vi "AnyThingToDoubleArray.vi"(0 "Claster":variant, 5 "Prefix":string, 11 "error in (no error)":errorcluster) -> (4 "NAME_ARR":string[](array[string]), 6 "DBL_ARR":dbl[](array[numeric]), 15 "error out":errorcluster)   [LabVIEW 2019]
uses:
  <vilib>/Utility/error.llb/Error Cluster From Error Code.vi
  <vilib>/ErrorRing/Error Ring.xnode
  <vilib>/Utility/Data Type/Type Definitions/Data Type.ctl
  <vilib>/Utility/Data Type/NI_Data Type.lvlib
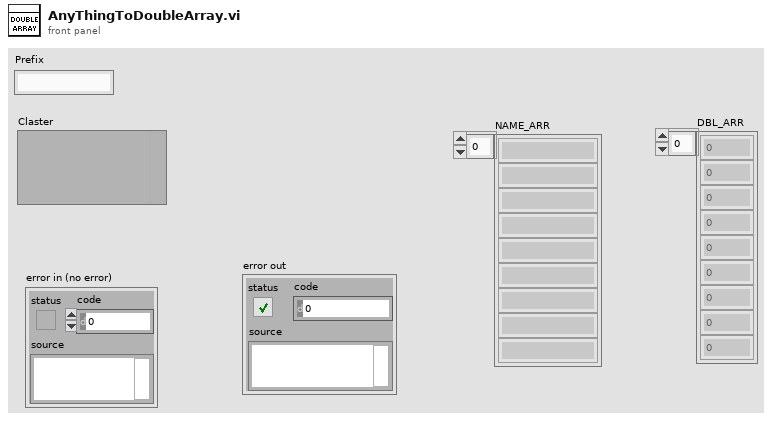
[diagram p1: front panel]
types:
  T1 = typedef "NI_Data Type.lvlib/Data Type.ctl" = enum8{"Invalid Type", "Void", "I8", "I16", "I32", "I64", "U8", "U16", "U32", "U64", "Single Float", "Double Float", "Extended Float", "Single Complex", "Double Complex", "Extended Complex", "Enum U8", "Enum U16", "Enum U32", "Enum U64", "Single Float With Unit", "Double Float With Unit", "Extended Float With Unit", "Single Complex with Unit", "Double Complex with Unit", "Extended Complex with Unit", "Boolean", "String", "Path", "Picture", "Tag", "Array", "Cluster", "Variant", "LV Variant", "Waveform", "Timestamp", "Digital Waveform", "Digital Data", "ExpressData", "Refnum", "External Data", "VI", "Poly VI", "LabVIEW Class Instance", "Fixed Point", "Set Collection", "Map Collection"}
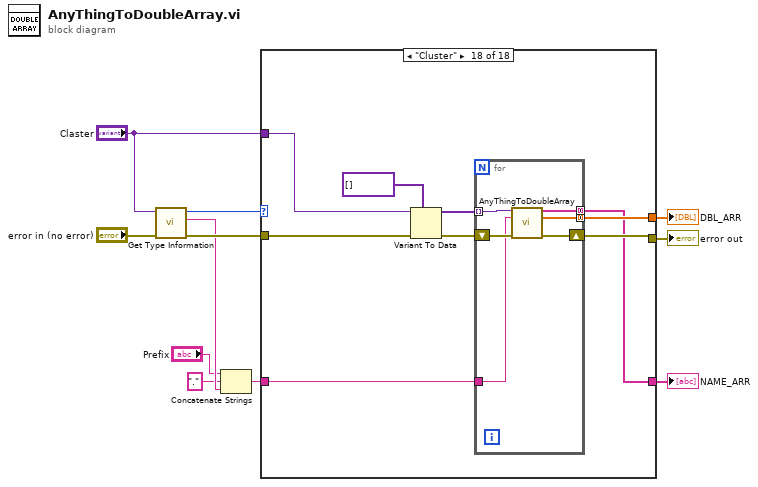
[diagram p0: block diagram]
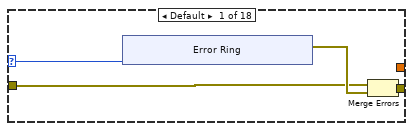
[diagram p2: hidden frame]
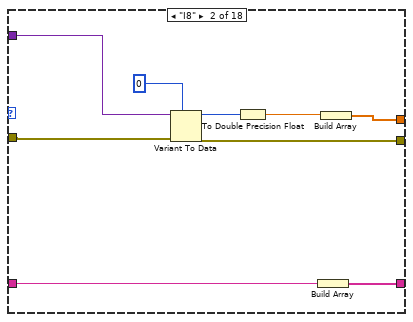
[diagram p3: hidden frame]
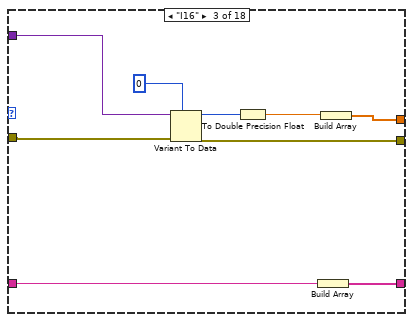
[diagram p4: hidden frame]
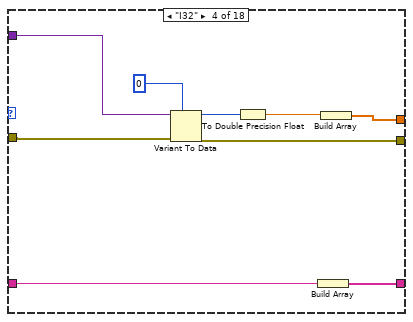
[diagram p5: hidden frame]
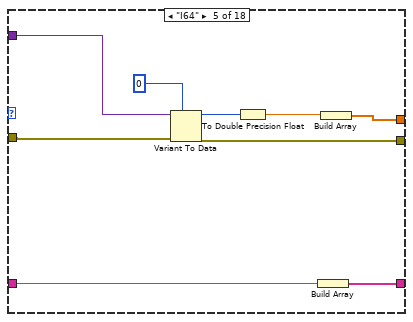
[diagram p6: hidden frame]
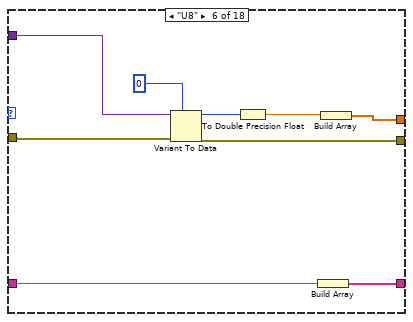
[diagram p7: hidden frame]
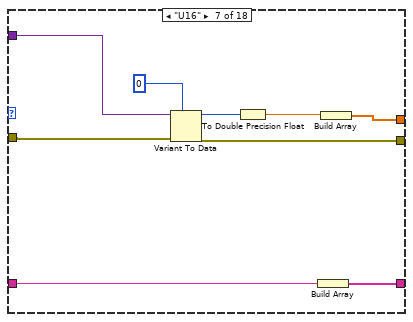
[diagram p8: hidden frame]
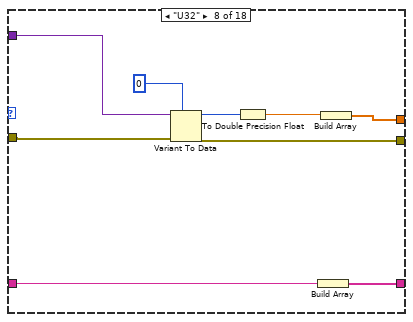
[diagram p9: hidden frame]
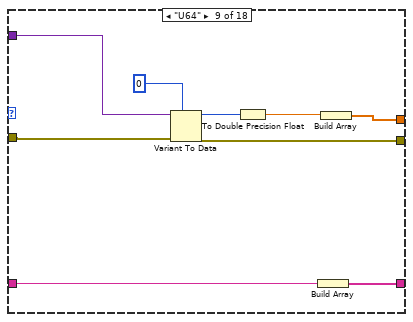
[diagram p10: hidden frame]
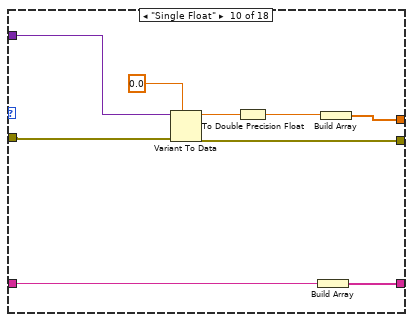
[diagram p11: hidden frame]
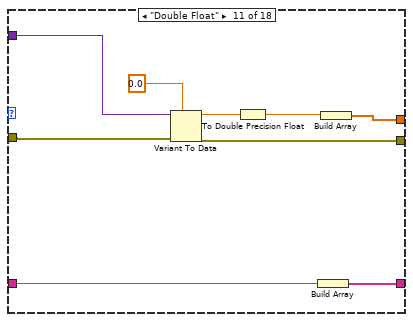
[diagram p12: hidden frame]
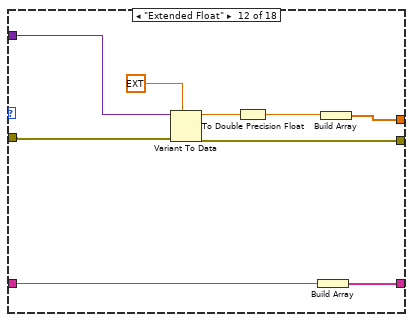
[diagram p13: hidden frame]
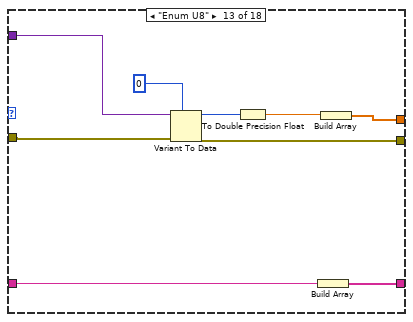
[diagram p14: hidden frame]
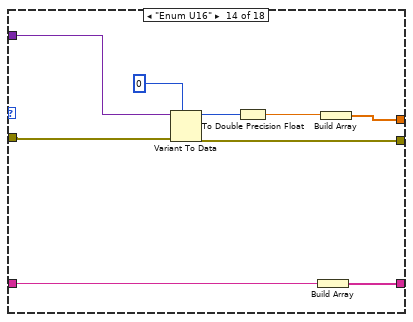
[diagram p15: hidden frame]
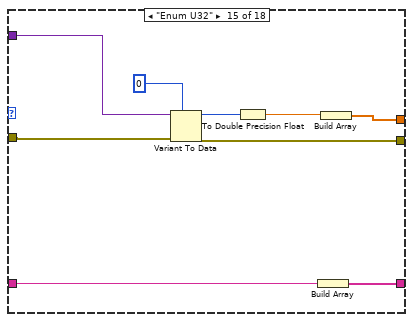
[diagram p16: hidden frame]
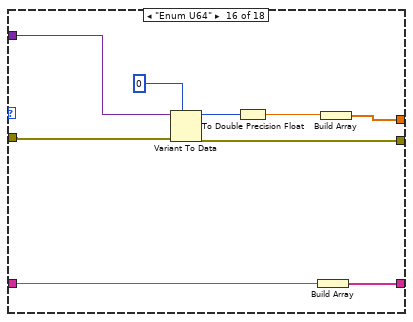
[diagram p17: hidden frame]
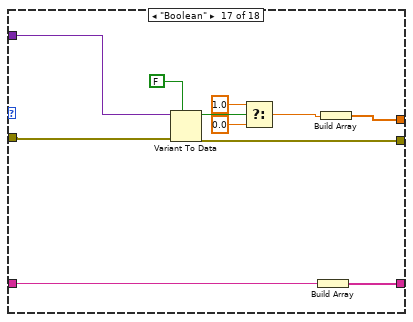
[diagram p18: hidden frame]
diagram:
  n1 = call <vilib>:"Get Type Information.vi"("error in (no error)"="error in (no error)", "variant"="Claster") -> ("error out"=w9:errorcluster, "name"=w5:string, "type"=w10:T1)  [unwired: 5 in, 2 out]
  n2 = Concatenate Strings("Prefix", "." ("string"), w5) -> (w3:string)
  n3 = case shown="\"Cluster\"" w10 {
    selector: w10 -> [w13 _ _ _ _ _ _ _ _ _ _ _ _ _ _ _ _ _]
    tunnel: w9 -> [w14 w31 w40 w49 w58 w67 w76 w85 w94 w103 w112 w121 w130 w139 w148 w157 w168 w173]
    tunnel: [w12 w26 w35 w44 w53 w62 w71 w80 w89 w98 w107 w116 w125 w134 w143 w152 w166 w176] -> w8
    tunnel: "Claster" -> [_ w30 w39 w48 w57 w66 w75 w84 w93 w102 w111 w120 w129 w138 w147 w156 w167 w171]
    tunnel: [_ w25 w34 w43 w52 w61 w70 w79 w88 w97 w106 w115 w124 w133 w142 w151 w165 w177] -> w6
    tunnel: w3 -> [_ w24 w33 w42 w51 w60 w69 w78 w87 w96 w105 w114 w123 w132 w141 w150 w164 w174]
    tunnel: [_ w23 w32 w41 w50 w59 w68 w77 w86 w95 w104 w113 w122 w131 w140 w149 w163 w175] -> w4
    frame Default {
      n4 = xnode "Error Ring"("parameter 0"=w13) -> ("error out"=w15:errorcluster)
      n5 = Merge Errors(w14, w15) -> (w12:errorcluster)
    }
    frame "I8" {
      n6 = Variant To Data(error in=w31, type=i8 0, Variant=w30) -> (data=w28:i8, error out=w26:errorcluster)
      n7 = To Double Precision Float(number=w28) -> (double precision float=w27:dbl)
      n8 = Build Array(w24) -> (w23:string[])
      n9 = Build Array(w27) -> (w25:dbl[])
    }
    frame "I16" {
      n10 = Variant To Data(error in=w40, type=i16 0, Variant=w39) -> (data=w37:i16, error out=w35:errorcluster)
      n11 = To Double Precision Float(number=w37) -> (double precision float=w36:dbl)
      n12 = Build Array(w33) -> (w32:string[])
      n13 = Build Array(w36) -> (w34:dbl[])
    }
    frame "I32" {
      n14 = Variant To Data(error in=w49, type=0, Variant=w48) -> (data=w46:i32, error out=w44:errorcluster)
      n15 = To Double Precision Float(number=w46) -> (double precision float=w45:dbl)
      n16 = Build Array(w42) -> (w41:string[])
      n17 = Build Array(w45) -> (w43:dbl[])
    }
    frame "I64" {
      n18 = Variant To Data(error in=w58, type=i64 0, Variant=w57) -> (data=w55:i64, error out=w53:errorcluster)
      n19 = To Double Precision Float(number=w55) -> (double precision float=w54:dbl)
      n20 = Build Array(w51) -> (w50:string[])
      n21 = Build Array(w54) -> (w52:dbl[])
    }
    frame "U8" {
      n22 = Variant To Data(error in=w67, type=u8 0, Variant=w66) -> (data=w64:u8, error out=w62:errorcluster)
      n23 = To Double Precision Float(number=w64) -> (double precision float=w63:dbl)
      n24 = Build Array(w60) -> (w59:string[])
      n25 = Build Array(w63) -> (w61:dbl[])
    }
    frame "U16" {
      n26 = Variant To Data(error in=w76, type=u16 0, Variant=w75) -> (data=w73:u16, error out=w71:errorcluster)
      n27 = To Double Precision Float(number=w73) -> (double precision float=w72:dbl)
      n28 = Build Array(w69) -> (w68:string[])
      n29 = Build Array(w72) -> (w70:dbl[])
    }
    frame "U32" {
      n30 = Variant To Data(error in=w85, type=u32 0, Variant=w84) -> (data=w82:u32, error out=w80:errorcluster)
      n31 = To Double Precision Float(number=w82) -> (double precision float=w81:dbl)
      n32 = Build Array(w78) -> (w77:string[])
      n33 = Build Array(w81) -> (w79:dbl[])
    }
    frame "U64" {
      n34 = Variant To Data(error in=w94, type=u64 0, Variant=w93) -> (data=w91:u64, error out=w89:errorcluster)
      n35 = To Double Precision Float(number=w91) -> (double precision float=w90:dbl)
      n36 = Build Array(w87) -> (w86:string[])
      n37 = Build Array(w90) -> (w88:dbl[])
    }
    frame "Single Float" {
      n38 = Variant To Data(error in=w103, type=sgl 0.0, Variant=w102) -> (data=w100:sgl, error out=w98:errorcluster)
      n39 = To Double Precision Float(number=w100) -> (double precision float=w99:dbl)
      n40 = Build Array(w96) -> (w95:string[])
      n41 = Build Array(w99) -> (w97:dbl[])
    }
    frame "Double Float" {
      n42 = Variant To Data(error in=w112, type=0.0, Variant=w111) -> (data=w109:dbl, error out=w107:errorcluster)
      n43 = To Double Precision Float(number=w109) -> (double precision float=w108:dbl)
      n44 = Build Array(w105) -> (w104:string[])
      n45 = Build Array(w108) -> (w106:dbl[])
    }
    frame "Extended Float" {
      n46 = Variant To Data(error in=w121, type=ext 0.0, Variant=w120) -> (data=w118:ext, error out=w116:errorcluster)
      n47 = To Double Precision Float(number=w118) -> (double precision float=w117:dbl)
      n48 = Build Array(w114) -> (w113:string[])
      n49 = Build Array(w117) -> (w115:dbl[])
    }
    frame "Enum U8" {
      n50 = Variant To Data(error in=w130, type=u8 0, Variant=w129) -> (data=w127:u8, error out=w125:errorcluster)
      n51 = To Double Precision Float(number=w127) -> (double precision float=w126:dbl)
      n52 = Build Array(w123) -> (w122:string[])
      n53 = Build Array(w126) -> (w124:dbl[])
    }
    frame "Enum U16" {
      n54 = Variant To Data(error in=w139, type=u16 0, Variant=w138) -> (data=w136:u16, error out=w134:errorcluster)
      n55 = To Double Precision Float(number=w136) -> (double precision float=w135:dbl)
      n56 = Build Array(w132) -> (w131:string[])
      n57 = Build Array(w135) -> (w133:dbl[])
    }
    frame "Enum U32" {
      n58 = Variant To Data(error in=w148, type=u32 0, Variant=w147) -> (data=w145:u32, error out=w143:errorcluster)
      n59 = To Double Precision Float(number=w145) -> (double precision float=w144:dbl)
      n60 = Build Array(w141) -> (w140:string[])
      n61 = Build Array(w144) -> (w142:dbl[])
    }
    frame "Enum U64" {
      n62 = Variant To Data(error in=w157, type=u64 0, Variant=w156) -> (data=w154:u64, error out=w152:errorcluster)
      n63 = To Double Precision Float(number=w154) -> (double precision float=w153:dbl)
      n64 = Build Array(w150) -> (w149:string[])
      n65 = Build Array(w153) -> (w151:dbl[])
    }
    frame "Boolean" {
      n66 = Variant To Data(error in=w168, type=FALSE, Variant=w167) -> (data=w161:bool, error out=w166:errorcluster)
      n67 = Select(t=1.0, s=w161, f=0.0) -> (s? t:f=w158:dbl)
      n68 = Build Array(w164) -> (w163:string[])
      n69 = Build Array(w158) -> (w165:dbl[])
    }
    frame "Cluster" {
      n70 = Variant To Data(error in=w173, type=variant[] [], Variant=w171) -> (data=w170:variant[], error out=w172:errorcluster)
      n71 = for {
        tunnel: w170 -> [w182] mode=indexing
        tunnel: [w181] -> w177 mode=concatenating
        shift-right: [w180] -> w176
        shift-left: w172 -> [w183]
        tunnel: [w179] -> w175 mode=concatenating
        tunnel: w174 -> [w178]
        n72 = call "AnyThingToDoubleArray.vi"("Claster"=w182, "Prefix"=w178, "error in (no error)"=w183) -> ("NAME_ARR"=w179:string[], "DBL_ARR"=w181:dbl[], "error out"=w180:errorcluster)  [unwired: 10 in]
      }
    }
  }
  "error out" <- w8
  "DBL_ARR" <- w6
  "NAME_ARR" <- w4
